vi "ProgMon.Create.vi"(8 "Error In":errorcluster, 10 "Ref CtrlEst":refnum<vi>, 11 "Ref CtrlComp":refnum<vi>) -> (0 "Error Out":errorcluster)   [LabVIEW 2024, in "EQMF.lvlib" / "Status Utils.lvlib"]
uses:
  Status Utils.lvlib
  Queues/Q.Element.ctl
  _Private/ProgMon.ProgMon Core.vi
  Queues/Queue Utils.lvlib
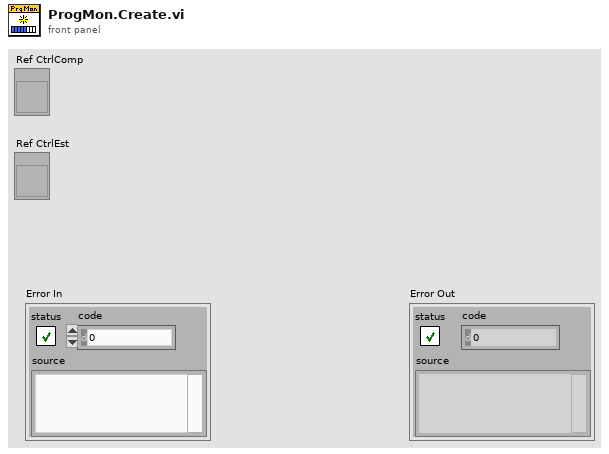
[diagram p1: front panel]
types:
  T1 = typedef "EQMF.lvlib/Queue Utils.lvlib/Q.Element.ctl" = cluster{"Cmd":string, "Sub":string, "Data1":variant, "Data2":variant}
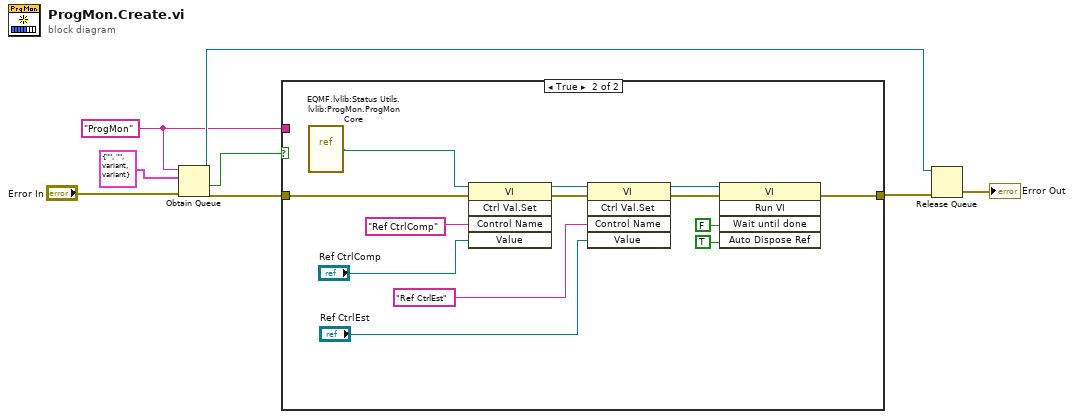
[diagram p0: block diagram]
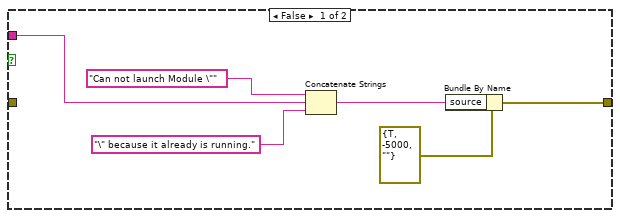
[diagram p2: hidden frame]
diagram:
  w1 = "ProgMon" ("Name [Do not use!]")
  n1 = Obtain Queue(name (unnamed)=w1, element data type=T1 {"Cmd"="", "Sub"="", "Data1"=variant, "Data2"=variant} ("MainQ.Element"), error in (no error)="Error In") -> (queue out=w4:refnum<queue>, created new?=w7:bool, error out=w5:errorcluster)  [unwired: 2 in]
  n2 = case shown="True" w7 {
    tunnel: w5 -> [_ w24]
    tunnel: [w12 w22] -> w6
    tunnel: w1 -> [w9 _]
    frame False {
      n3 = Concatenate Strings("Can not launch Module \"", w9, "\" because it already is running.") -> (w10:string)
      n4 = Bundle By Name(cluster=errorcluster {"status"=TRUE, "code"=-5000, "source"=""} ("error constant"), "source"=w10) -> (w12:errorcluster)
    }
    frame True {
      n5 = vi-ref "EQMF.lvlib:Status Utils.lvlib:ProgMon.ProgMon Core.vi"() -> (w23:refnum<vi>)
      n6 = invoke class="VI" method="Ctrl Val.Set"(reference=w23, error in=w24, "Control Name"="Ref CtrlComp", "Value"="Ref CtrlComp") -> (reference out=w21:refnum<vi>, error out=w20:errorcluster)  [unwired: 1 in, 3 out]
      n7 = invoke class="VI" method="Ctrl Val.Set"(reference=w21, error in=w20, "Control Name"="Ref CtrlEst", "Value"="Ref CtrlEst") -> (reference out=w19:refnum<vi>, error out=w18:errorcluster)  [unwired: 1 in, 3 out]
      n8 = invoke class="VI" method="Run VI"(reference=w19, error in=w18, "Wait until done"=FALSE ("Wait Until Done"), "Auto Dispose Ref"=TRUE ("Auto Dispose Reference")) -> (error out=w22:errorcluster)  [unwired: 1 in, 4 out]
    }
  }
  n9 = Release Queue(queue=w4, error in (no error)=w6) -> (error out=→"Error Out":errorcluster)  [unwired: 1 in, 2 out]
